vi "CRYGet Channel Infor Table.vi"(9 "Channel Name":string, 10 "Input/Output?":bool=TRUE, 11 "Hardware In":string) -> (0 "Digital/Analog":bool, 1 "SoundCard Unit":string, 3 "List Item Out":string[][](array[string]))   [LabVIEW 2013]
uses:
  CRYMainGlobal.vi
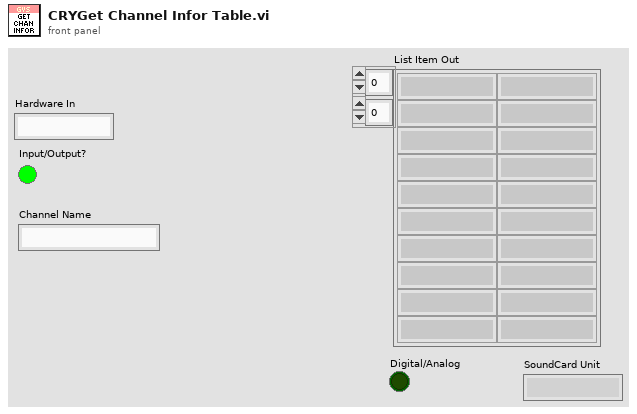
[diagram p1: front panel]
types:
  T1 = typedef "CRYHardware Channel Info.ctl" = cluster{"ID":i32, "Name":string, "Digital":bool, "Input":bool, "Device Name":string, "Hardware Ch ID":u8, "Vmax (V)":dbl, "Latency (samples)":dbl, "Sampling Rate (Hz)":u32, "Bit Depth":u32, "Anti-aliasing Factor (%fs)":sgl, "DAQmx Channel":tag, "term config":i32, "Coupling":i32, "IEPE en":bool, "ASIOChannel Name":string, "Audio Driver":u16, "ASIOChannel Index":u8}
  T2 = enum32{"English", "Chinese", "Korean", "Japanese", "Russian", "Chinese traditional"}
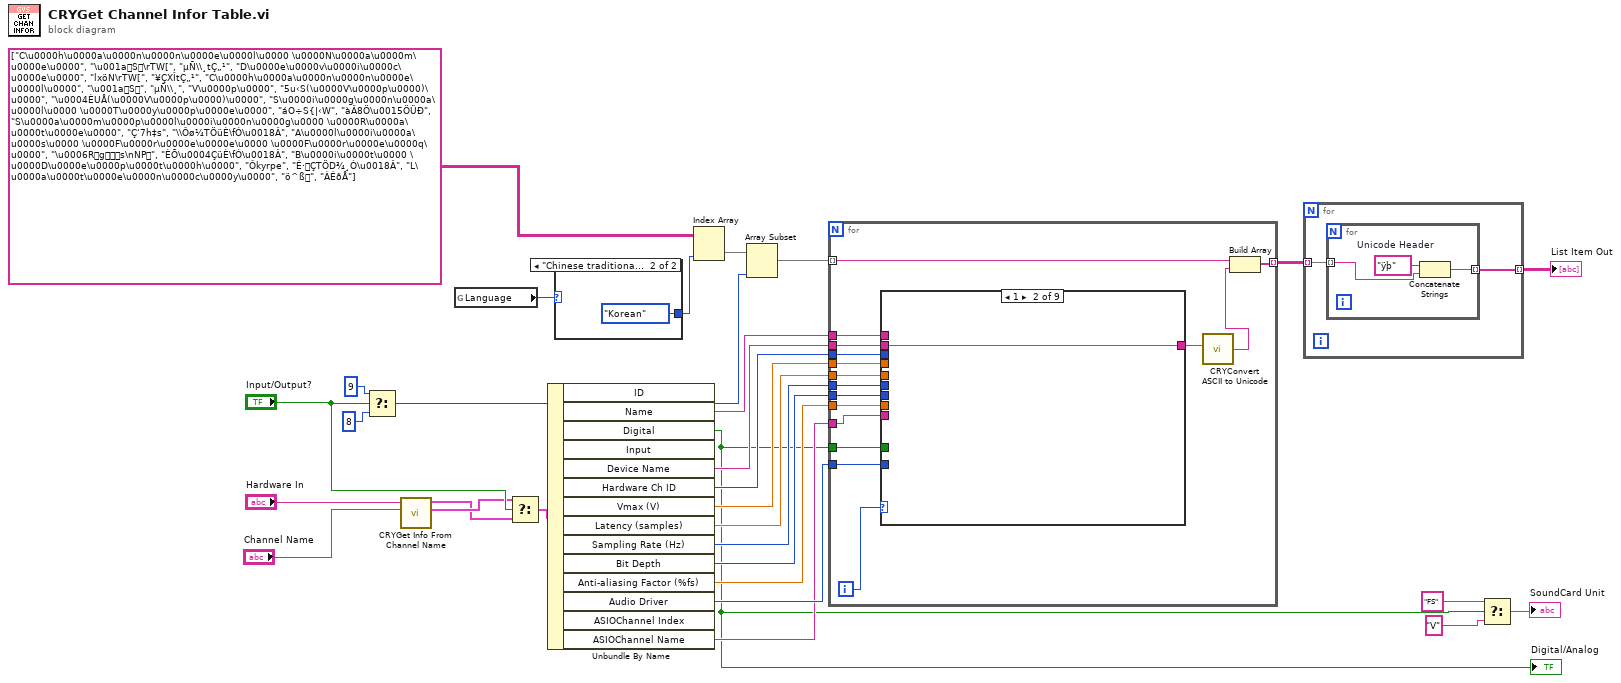
[diagram p0: block diagram]
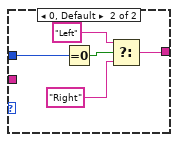
[diagram p4: hidden frame]
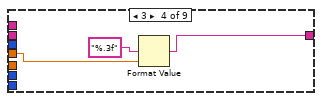
[diagram p5: hidden frame]
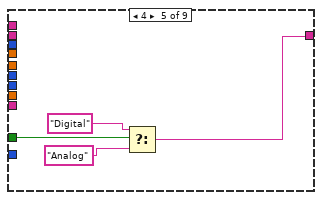
[diagram p6: hidden frame]
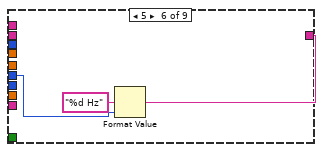
[diagram p7: hidden frame]
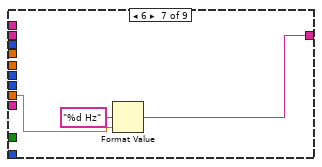
[diagram p8: hidden frame]
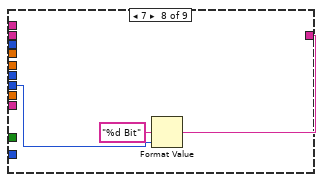
[diagram p9: hidden frame]
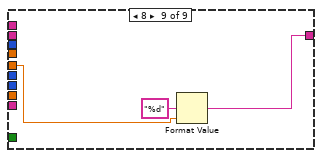
[diagram p10: hidden frame]
diagram:
  n1 = Select(t=9 ("index"), s="Input/Output?", f=8 ("index")) -> (s? t:f=w24:i32)
  n2 = call "CRYGet Info From Channel Name.vi"("Channel Name"="Channel Name", "Hardware In"="Hardware In") -> ("In_ChannelInfo"=w20:T1, "Out_ChannelInfo"=w19:T1)  [unwired: 8 in]
  n3 = global read "CRYMainGlobal.vi" "Language"() -> (w30:T2)
  n4 = Select(t=w20, s="Input/Output?", f=w19) -> (s? t:f=w18:T1)
  n5 = Unbundle By Name(w18) -> ("Name"=w16:string, "Digital"=w4:bool, "Device Name"=w15:string, "Hardware Ch ID"=w14:u8, "Vmax (V)"=w13:dbl, "Latency (samples)"=w12:dbl, "Sampling Rate (Hz)"=w11:u32, "Bit Depth"=w10:u32, "Anti-aliasing Factor (%fs)"=w9:sgl, "Audio Driver"=w6:u16, "ASIOChannel Name"=w5:string)  [unwired: 3 out]
  "Digital/Analog" <- w4
  n6 = case shown="\"Chinese traditional\"" w30 {
    selector: w30 -> [w31 _]
    tunnel: [w31 T2."Korean" ("Language")] -> w29
    frame "English", Default {
    }
    frame "Chinese traditional" {
    }
  }
  n7 = Index Array(array=string[][] [["C\u0000h\u0000a\u0000n\u0000n\u0000e\u0000l\u0000 \u0000N\u0000a\u0000m\u0000e\u0000", "\u001aS\rTW[", "µÑ\\¸tÇ„¹"], ["D\u0000e\u0000v\u0000i\u0000c\u0000e\u0000", "lxöN\rTW[", "¥ÇXÎtÇ„¹"], ["C\u0000h\u0000a\u0000n\u0000n\u0000e\u0000l\u0000", "\u001aS", "µÑ\\¸"], ["V\u0000p\u0000", "5u‹S(\u0000V\u0000p\u0000)\u0000", "\u0004ÈUÅ(\u0000V\u0000p\u0000)\u0000"], ["S\u0000i\u0000g\u0000n\u0000a\u0000l\u0000 \u0000T\u0000y\u0000p\u0000e\u0000", "áO÷S{|‹W", "àÂ8Ö\u0015ÖÜÐ"], ["S\u0000a\u0000m\u0000p\u0000l\u0000i\u0000n\u0000g\u0000 \u0000R\u0000a\u0000t\u0000e\u0000", "Ç‘7h‡s", "\\Ôø¼TÖüÈ\fÓ\u0018Â"], ["A\u0000l\u0000i\u0000a\u0000s\u0000 \u0000F\u0000r\u0000e\u0000e\u0000 \u0000F\u0000r\u0000e\u0000q\u0000", "\u0006Rgs\nNP", "ÈÕ\u0004ÇüÈ\fÓ\u0018Â"], ["B\u0000i\u0000t\u0000 \u0000D\u0000e\u0000p\u0000t\u0000h\u0000", "Ôkyrpe", "É·ÇTÖD¾¸Ò\u0018Â"], ["L\u0000a\u0000t\u0000e\u0000n\u0000c\u0000y\u0000", "ö^ß", "ÀÉðÅ"]] ("Item Names"), index (col)=w29) -> (element=w25:string[])  [unwired: 1 in]
  n8 = Array Subset(array=w25, length=w24) -> (w17:string[])  [unwired: 1 in]
  n9 = for {
    tunnel: w17 -> [w48] mode=indexing
    tunnel: [w47] -> w8 mode=indexing
    tunnel: w16 -> [w45]
    tunnel: w15 -> [w44]
    tunnel: w14 -> [w43]
    tunnel: w13 -> [w42]
    tunnel: w12 -> [w41]
    tunnel: w11 -> [w40]
    tunnel: w10 -> [w39]
    tunnel: w4 -> [w38]
    tunnel: w9 -> [w37]
    tunnel: w6 -> [w34]
    tunnel: w5 -> [w33]
    i -> [w46]
    n10 = case shown="1" w46 {
      tunnel: w45 -> [w49 _ _ _ _ _ _ _ _]
      tunnel: [w49 w50 w53 w61 w64 w68 w72 w74 w77] -> w36
      tunnel: w44 -> [_ w50 _ _ _ _ _ _ _]
      tunnel: w43 -> [_ _ w54 _ _ _ _ _ _]
      tunnel: w42 -> [_ _ _ w63 _ _ _ _ _]
      tunnel: w41 -> [_ _ _ _ _ _ _ _ w78]
      tunnel: w40 -> [_ _ _ _ _ w69 _ _ _]
      tunnel: w39 -> [_ _ _ _ _ _ _ w75 _]
      tunnel: w38 -> [_ _ _ _ w67 _ _ _ _]
      tunnel: w37 -> [_ _ _ _ _ _ w71 _ _]
      tunnel: w34 -> [_ _ w52 _ _ _ _ _ _]
      tunnel: w33 -> [_ _ w51 _ _ _ _ _ _]
      frame 0, Default {
      }
      frame 1 {
      }
      frame 2 {
        n11 = case shown="2" w52 {
          tunnel: w54 -> [_ w60]
          tunnel: [w55 w56] -> w53
          tunnel: w51 -> [w55 _]
          frame 2 {
          }
          frame 0, Default {
            n12 = Equal To 0?(x=w60) -> (x = 0?=w59:bool)
            n13 = Select(t="Left" ("Name"), s=w59, f="Right" ("Name")) -> (s? t:f=w56:string)
          }
        }
      }
      frame 3 {
        n14 = Format Value(format string="%.3f", value (0)=w63) -> (output string=w61:string)  [unwired: 1 in]
      }
      frame 4 {
        n15 = Select(t="Digital" ("output string"), s=w67, f="Analog" ("output string")) -> (s? t:f=w64:string)
      }
      frame 5 {
        n16 = Format Value(format string="%d Hz", value (0)=w69) -> (output string=w68:string)  [unwired: 1 in]
      }
      frame 6 {
        n17 = Format Value(format string="%d Hz", value (0)=w71) -> (output string=w72:string)  [unwired: 1 in]
      }
      frame 7 {
        n18 = Format Value(format string="%d Bit", value (0)=w75) -> (output string=w74:string)  [unwired: 1 in]
      }
      frame 8 {
        n19 = Format Value(format string="%d", value (0)=w78) -> (output string=w77:string)  [unwired: 1 in]
      }
    }
    n20 = call "CRYConvert ASCII to Unicode.vi"("ASCII"=w36) -> ("Unicode"=w35:string)  [unwired: 4 in]
    n21 = Build Array(w48, w35) -> (w47:string[])
  }
  n22 = for {
    tunnel: w8 -> [w81] mode=indexing
    tunnel: [w80] -> w7 mode=indexing
    n23 = for {
      tunnel: w81 -> [w83] mode=indexing
      tunnel: [w82] -> w80 mode=indexing
      w84 = "ÿþ"  # Unicode Header
      n24 = Concatenate Strings(w84, w83) -> (w82:string)
    }
  }
  "List Item Out" <- w7
  n25 = Select(t="FS", s=w4, f="V") -> (s? t:f=→"SoundCard Unit":string)
